vi "Read Configuration Class.vi"(8 "error in (no error)":errorcluster, 11 "Instrument in":refnum<class "Instrument.lvclass">) -> (0 "error out":errorcluster, 2 "Configuration":refnum<class "Configuration.lvclass">, 3 "Instrument out":refnum<class "Instrument.lvclass">)   [LabVIEW 2019, in "Instrument.lvlib" / "Instrument.lvclass"]
uses:
  Instrument.lvclass
  C:/Program Files (x86)/National Instruments/LabVIEW 2019/vi.lib/JKI/JKI SMO/SMO/SMO.lvclass
  <userlib>/LevyLab/Configuration/Configuration.lvclass
  Instrument.lvclass/Instrument.ctl
  <userlib>/LevyLab/Configuration/Configuration.lvclass/Configuration.ctl
  <vilib>/JKI/JKI SMO/SMO/SMO.lvclass
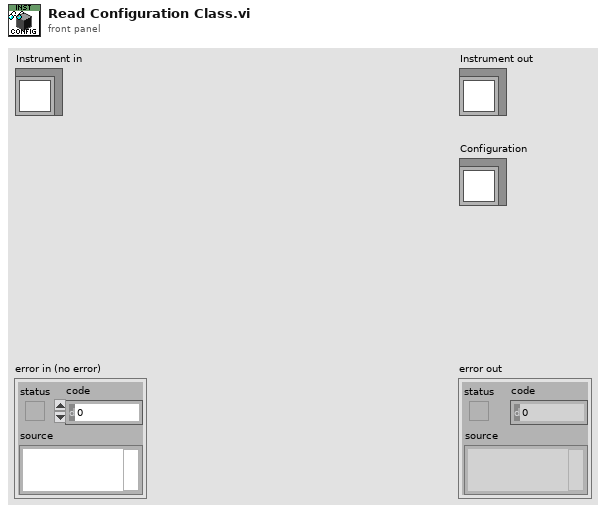
[diagram p1: front panel]
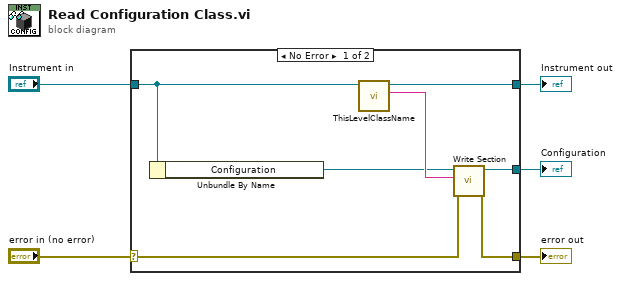
[diagram p0: block diagram]
diagram:
  n1 = case shown="No Error" "error in (no error)" {
    selector: "error in (no error)" -> [w9 w13]
    tunnel: [w8 w13] -> w4
    tunnel: [w7 w14] -> w2
    tunnel: "Instrument in" -> [w6 w14]
    tunnel: [w10 _] -> w1
    frame No Error {
      n2 = Unbundle By Name(w6) -> ("Configuration"=w11:refnum<class "Configuration.lvclass">)
      n3 = call <vilib>:"ThisLevelClassName.vi"("SMO"=w6) -> ("Level class name"=w12:string, "SMO out"=w7:refnum<class "Instrument.lvclass">)  [unwired: 9 in]
      n4 = call <userlib>:"Write Section.vi"("error in (no error)"=w9, "Section"=w12, "Configuration in"=w11) -> ("error out"=w8:errorcluster, "Configuration out"=w10:refnum<class "Configuration.lvclass">)  [unwired: 7 in]
    }
    frame Error {
    }
  }
  "error out" <- w4
  "Instrument out" <- w2
  "Configuration" <- w1
